vi "Open.vi"(7 "Allow multiple opens?":bool, 8 "error in (no error)":errorcluster, 10 "Channel Names":tag[](array[tag])) -> (0 "error out":errorcluster, 3 "DIO Ref Out":T1)   [LabVIEW 2021, in "DIO.lvlib"]
doc: "Opens a reference to one or more digital I/O channels. You must open a reference before you read or write values."
uses:
  <vilib>/myRIO/Instrument Drivers/Onboard IO/DIO/DIO.lvlib
  <vilib>/myRIO/Instrument Drivers/Onboard IO/DIO/typedefs/DIO Reference.ctl
  <vilib>/myRIO/Common/Instrument Driver Framework/Utilities/typedefs/myRIO Generic Hardware Reference.ctl
  <vilib>/myRIO/Common/Instrument Driver Framework/Utilities/typedefs/Hardware Version Enum.ctl
  <vilib>/myRIO/Common/Instrument Driver Framework/Utilities/typedefs/myRIO v1.0 Reference.ctl
  <vilib>/myRIO/Common/Instrument Driver Framework/Utilities/typedefs/Generic FPGA Reference.ctl
  <vilib>/myRIO/Common/Instrument Driver Framework/myRIO v1.0/DIO/typedefs/DIO Channels List.ctl
  <vilib>/myRIO/Common/Instrument Driver Framework/myRIO v1.0/DIO/typedefs/DIO Channels Enum.ctl
  <vilib>/myRIO/Common/Instrument Driver Framework/Utilities/vis/Validate Channels.vi
  <vilib>/myRIO/Common/Instrument Driver Framework/myRIO v1.0/DIO/vis/myRIO v1.0 Reserve DIO.vi
  <vilib>/myRIO/Common/Instrument Driver Framework/roboRIO v1.0/DIO/vis/roboRIO v1.0 Reserve DIO.vi
  <vilib>/myRIO/Common/Instrument Driver Framework/ELVIS III v1.0/DIO/vis/ELVIS III v1.0 Reserve DIO.vi
  <vilib>/myRIO/Common/Instrument Driver Framework/myRIO v1.0/Resource Manager/vis/myRIO v1.0 Reserve Channel List.vi
  <vilib>/myRIO/Common/Instrument Driver Framework/myRIO v1.0/DIO/vis/myRIO v1.0 Build MUX Configuration DIO.vi
  <vilib>/myRIO/Common/Instrument Driver Framework/roboRIO v1.0/DIO/vis/roboRIO v1.0 Build MUX Configuration DIO.vi
  <vilib>/myRIO/Common/Instrument Driver Framework/roboRIO v1.0/Resource Manager/vis/roboRIO v1.0 Reserve Channel List.vi
  <vilib>/myRIO/Common/Instrument Driver Framework/ELVIS III v1.0/DIO/vis/ELVIS III v1.0 Build MUX Configuration DIO.vi
  <vilib>/myRIO/Common/Instrument Driver Framework/myRIO v1.0/Resource Manager/vis/myRIO v1.0 Reserve Channel.vi
  <vilib>/myRIO/Common/Instrument Driver Framework/myRIO v1.0/Resource Manager/vis/myRIO v1.0 Unreserve Channel.vi
  <vilib>/myRIO/Common/Instrument Driver Framework/myRIO v1.0/Resource Manager/vis/myRIO v1.0 Create Configuration List.vi
  <vilib>/myRIO/Common/Instrument Driver Framework/roboRIO v1.0/Resource Manager/vis/roboRIO v1.0 Create Configuration List.vi
  <vilib>/myRIO/Common/Instrument Driver Framework/roboRIO v1.0/Resource Manager/vis/roboRIO v1.0 Reserve Channel.vi
  <vilib>/myRIO/Common/Instrument Driver Framework/roboRIO v1.0/Resource Manager/vis/roboRIO v1.0 Unreserve Channel.vi
  <vilib>/myRIO/Common/Instrument Driver Framework/ELVIS III v1.0/Resource Manager/vis/ELVIS III v1.0 Create Configuration List.vi
  <vilib>/myRIO/Common/Instrument Driver Framework/myRIO v1.0/Resource Manager/vis/myRIO v1.0 Build Mutex Name.vi
  <vilib>/myRIO/Common/Instrument Driver Framework/roboRIO v1.0/Resource Manager/vis/roboRIO v1.0 Build Mutex Name.vi
  <vilib>/Utility/VariantDataType/GetNumericInfo.vi
  <vilib>/myRIO/Common/Instrument Driver Framework/Utilities/vis/IO Manager.vi
  <vilib>/myRIO/Common/Instrument Driver Framework/Utilities/vis/Configuration Manager.vi
  <vilib>/myRIO/Common/Instrument Driver Framework/myRIO v1.0/Resource Manager/vis/myRIO v1.0 Configure IO.vi
  <vilib>/myRIO/Common/Instrument Driver Framework/myRIO v1.0/myRIO v1.0 Close.vi
  <vilib>/myRIO/Common/Instrument Driver Framework/roboRIO v1.0/Resource Manager/vis/roboRIO v1.0 Configure IO.vi
  <vilib>/myRIO/Common/Instrument Driver Framework/ELVIS III v1.0/Resource Manager/vis/ELVIS III v1.0 Reserve Channel List.vi
  <vilib>/myRIO/Common/Instrument Driver Framework/ELVIS III v1.0/Resource Manager/vis/ELVIS III v1.0 Configure IO.vi
  <vilib>/userdefined/High Color/nirio_resource_hc.ctl
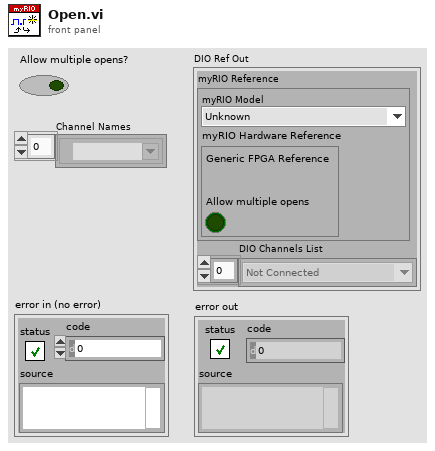
[diagram p1: front panel]
types:
  T1 = typedef "DIO.lvlib/DIO Reference.ctl" = cluster{"myRIO Reference":T2, "DIO Channels List":T6}
  T2 = typedef "myRIO Generic Hardware Reference.ctl" = cluster{"myRIO Model":T3, "myRIO Hardware Reference":T4}
  T3 = typedef "Hardware Version Enum.ctl" = enum16{"Unknown", "myRIO-1900", "myRIO-1950", "roboRIO", "NI ELVIS RIO CM", "ELVIS III"}
  T4 = typedef "myRIO v1.0 Reference.ctl" = cluster{"Generic FPGA Reference":T5, "Allow multiple opens":bool}
  T5 = typedef "Generic FPGA Reference.ctl" = refnum<k20>
  T6 = typedef "DIO Channels List.ctl" = T7[]
  T7 = typedef "DIO Channels Enum.ctl" = enum16{"Not Connected", "C/DIO0", "C/DIO1", "C/DIO2", "C/DIO3", "C/DIO4", "C/DIO5", "C/DIO6", "C/DIO7", "A/DIO0", "A/DIO1", "A/DIO2", "A/DIO3", "A/DIO4", "A/DIO5", "A/DIO6", "A/DIO7", "A/DIO8", "A/DIO9", "A/DIO10", "A/DIO11", "A/DIO12", "A/DIO13", "A/DIO14", "A/DIO15", "A/DIO16", "A/DIO17", "A/DIO18", "A/DIO19", "B/DIO0", "B/DIO1", "B/DIO2", "B/DIO3", "B/DIO4", "B/DIO5", "B/DIO6", "B/DIO7", "B/DIO8", "B/DIO9", "B/DIO10", "B/DIO11", "B/DIO12", "B/DIO13", "B/DIO14", "B/DIO15", "B/DIO16", "B/DIO17", "B/DIO18", "B/DIO19", "LED0", "LED1", "LED2", "LED3", "Button0", "DIO/DIO0", "DIO/DIO1", "DIO/DIO2", "DIO/DIO3", "DIO/DIO4", "DIO/DIO5", "DIO/DIO6", "DIO/DIO7", "DIO/DIO8", "DIO/DIO9", "SPI/CS0", "SPI/CS1", "SPI/CS2", "SPI/CS3", "LED RADIO (Green)", "LED RADIO (Red)", "LED COMM (Green)", "LED COMM (Red)", "LED MODE (Green)", "LED MODE (Red)"}
  T8 = typedef "nirio_resource_hc.ctl" = tag
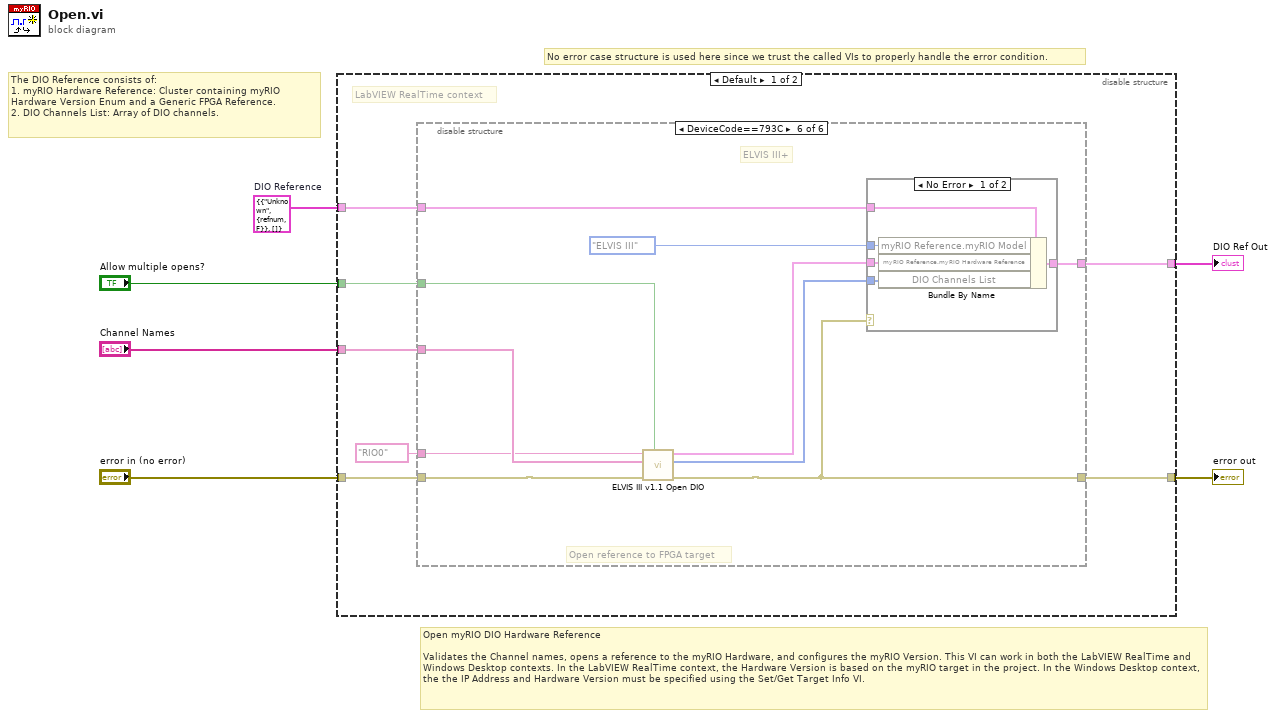
[diagram p0: block diagram]
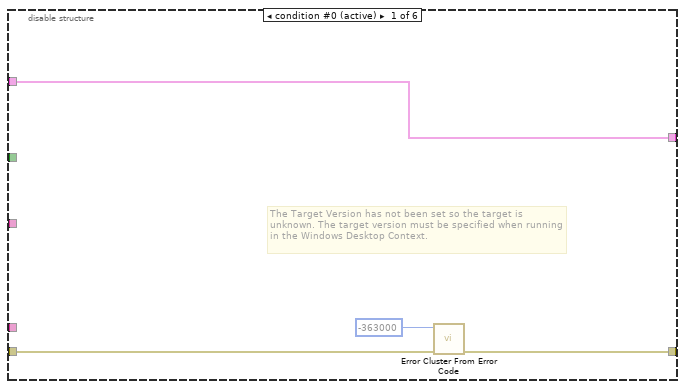
[diagram p2: hidden frame]
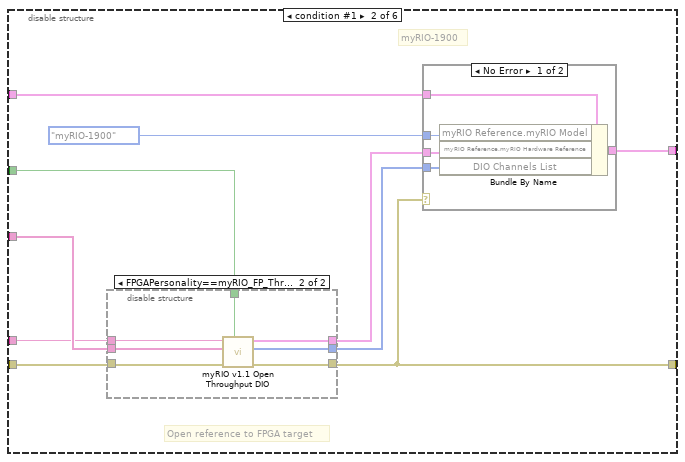
[diagram p3: hidden frame]
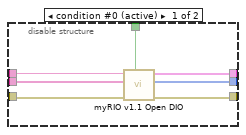
[diagram p4: hidden frame]
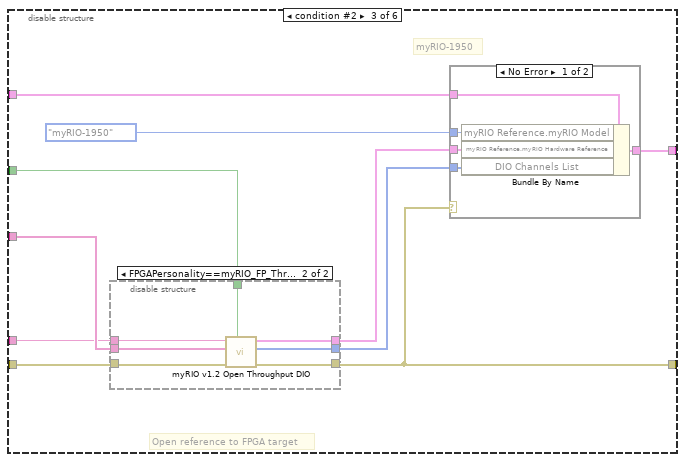
[diagram p6: hidden frame]
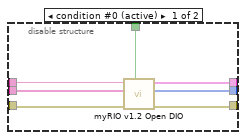
[diagram p7: hidden frame]
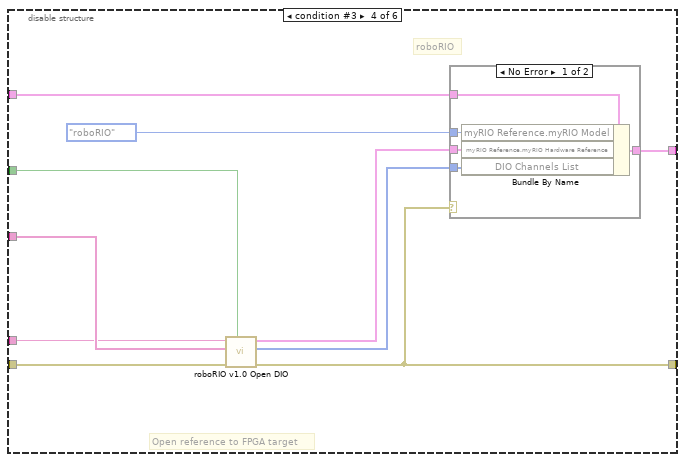
[diagram p9: hidden frame]
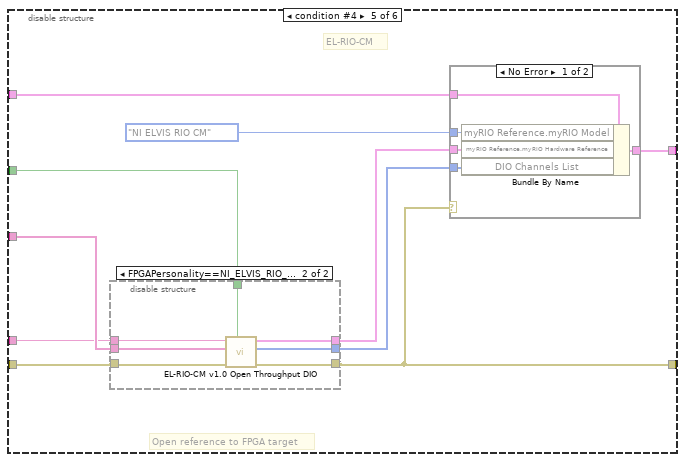
[diagram p11: hidden frame]
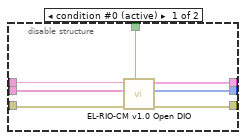
[diagram p12: hidden frame]
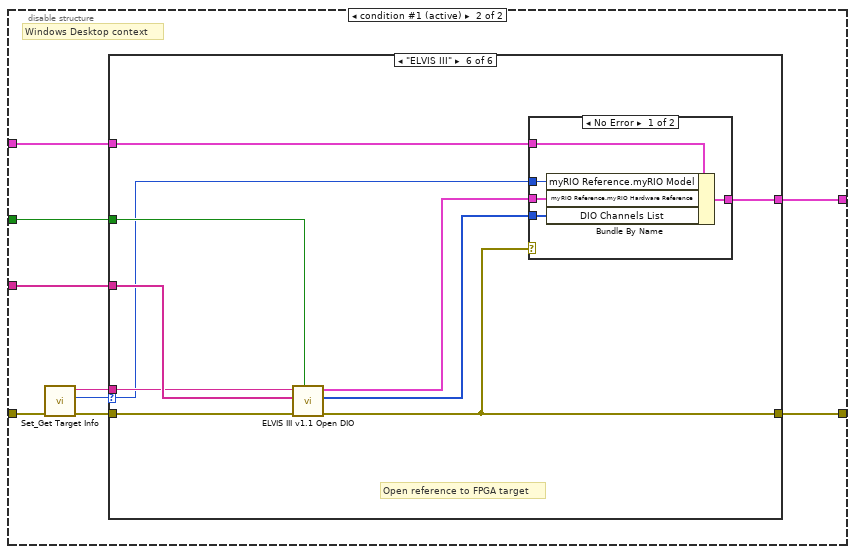
[diagram p15: hidden frame]
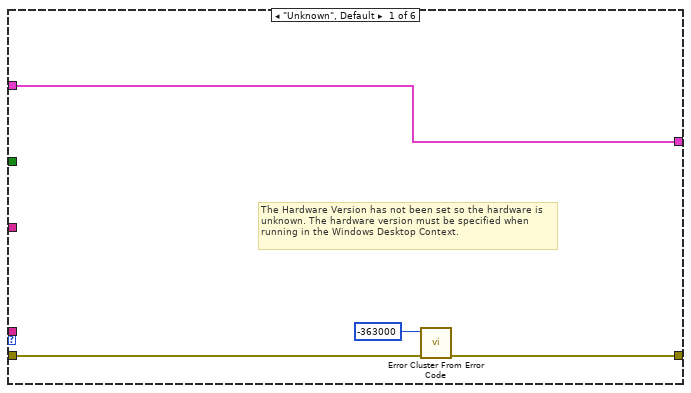
[diagram p16: hidden frame]
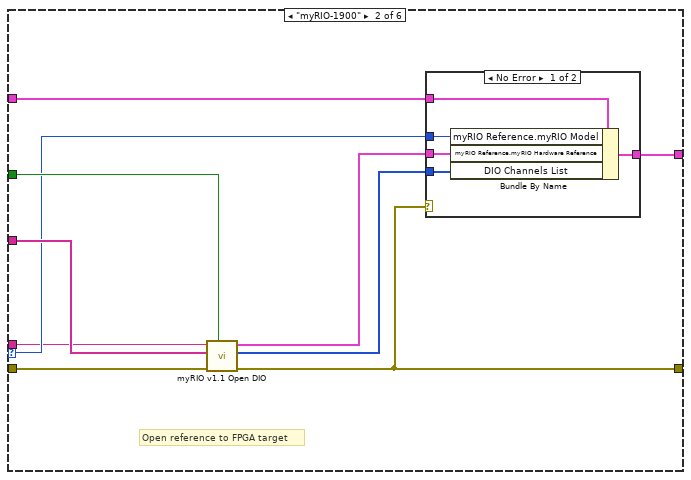
[diagram p17: hidden frame]
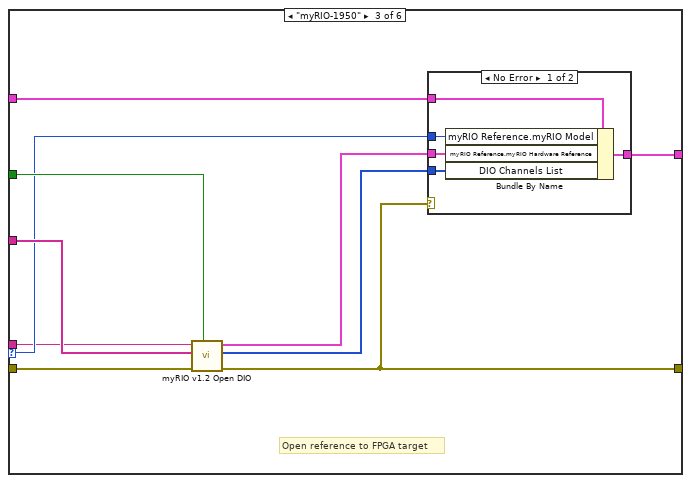
[diagram p19: hidden frame]
diagram:
  w3 = T1 {"myRIO Reference"={"myRIO Model"=enum."Unknown", "myRIO Hardware Reference"={"Generic FPGA Reference"=refnum, "Allow multiple opens"=FALSE}}, "DIO Channels List"=[]}  # DIO Reference
  # "Open myRIO DIO Hardware Reference\n\nValidates the Channel names, opens a reference to the myRIO Hardware, and configures the myRIO Version. This VI can work in both the LabVIEW RealTime and Windows Desktop contexts. In the LabVIEW RealTime context, the Hardware Version is based on the myRIO target in the project. In the Windows Desktop context, the the IP Address and Hardware Version must be specified using the Set/Get Target Info VI."
  # "No error case structure is used here since we trust the called VIs to properly handle the error condition."
  # "The DIO Reference consists of:\n1. myRIO Hardware Reference: Cluster containing myRIO Hardware Version Enum and a Generic FPGA Reference.\n2. DIO Channels List: Array of DIO channels."
  n1 = disable-structure shown="Default" {
    disable-tunnel: [w13 w147] -> w6
    disable-tunnel: "Channel Names" -> [w12 w144]
    disable-tunnel: "Allow multiple opens?" -> [w11 w146]
    disable-tunnel: [w10 w145] -> w2
    disable-tunnel: "error in (no error)" -> [w9 w143]
    disable-tunnel: w3 -> [w8 w142]
    frame condition #0 {
      # "LabVIEW RealTime context"
      n2 = disable-structure shown="DeviceCode==793C" {
        disable-tunnel: [w17 w18 w48 w78 w100 w125] -> w13
        disable-tunnel: w12 -> [_ w27 w57 w87 w96 w128]
        disable-tunnel: w11 -> [_ w22 w56 w86 w94 w129]
        disable-tunnel: [w14 w26 w55 w85 w103 w124] -> w10
        disable-tunnel: w9 -> [w16 w24 w53 w83 w97 w126]
        disable-tunnel: w8 -> [w14 w21 w51 w81 w101 w130]
        disable-tunnel: T8 "RIO0" ("Resource name") -> [_ w19 w49 w79 w95 w127]
        frame condition #0 (active) {
          # "The Target Version has not been set so the target is unknown. The target version must be specified when running in the Windows Desktop Context."
          n3 = call <vilib>:"Error Cluster From Error Code.vi"("error in (no error)"=w16, "error code (0)"=-363000) -> ("error out"=w17:errorcluster)  [unwired: 7 in]
        }
        frame condition #1 {
          # "myRIO-1900"
          # "Open reference to FPGA target"
          n4 = disable-structure shown="FPGAPersonality==myRIO_FP_Throughput" {
            disable-tunnel: w27 -> [w34 w41]
            disable-tunnel: w24 -> [w33 w40]
            disable-tunnel: [w32 w39] -> w23
            disable-tunnel: w22 -> [w31 w38]
            disable-tunnel: [w30 w37] -> w20
            disable-tunnel: w19 -> [w29 w36]
            disable-tunnel: [w28 w35] -> w18
            frame condition #0 (active) {
              n5 = call <vilib>:"myRIO v1.1 Open DIO.vi"("Allow multiple opens?"=w31, "error in (no error)"=w33, "Channel Names"=w34, "Resource name"=w29) -> ("error out"=w28:errorcluster, "DIO Channel List"=w30:T6, "myRIO Ref Out"=w32:T4)  [unwired: 5 in]
            }
            frame condition #1 {
              n6 = call <vilib>:"myRIO v1.1 Open Throughput DIO.vi"("Allow multiple opens?"=w38, "error in (no error)"=w40, "Channel Names"=w41, "Resource name"=w36) -> ("error out"=w35:errorcluster, "DIO Channel List"=w37:T6, "myRIO Ref Out"=w39:T4)  [unwired: 5 in]
            }
          }
          n7 = case shown="No Error" w18 {
            tunnel: [w46 w47] -> w26
            tunnel: Hardware_Version_Enum."myRIO-1900" ("Hardware Version Enum") -> [w45 _]
            tunnel: w23 -> [w42 _]
            tunnel: w21 -> [w44 w47]
            tunnel: w20 -> [w43 _]
            frame No Error {
              n8 = Bundle By Name(cluster=w44, "myRIO Reference.myRIO Model"=w45, "myRIO Reference.myRIO Hardware Reference"=w42, "DIO Channels List"=w43) -> (w46:T1)
            }
            frame Error {
            }
          }
        }
        frame condition #2 {
          # "myRIO-1950"
          # "Open reference to FPGA target"
          n9 = disable-structure shown="FPGAPersonality==myRIO_FP_Throughput" {
            disable-tunnel: w57 -> [w64 w71]
            disable-tunnel: w56 -> [w63 w70]
            disable-tunnel: w53 -> [w62 w69]
            disable-tunnel: [w61 w68] -> w52
            disable-tunnel: [w60 w67] -> w50
            disable-tunnel: w49 -> [w59 w66]
            disable-tunnel: [w58 w65] -> w48
            frame condition #0 (active) {
              n10 = call <vilib>:"myRIO v1.2 Open DIO.vi"("Allow multiple opens?"=w63, "error in (no error)"=w62, "Channel Names"=w64, "Resource name"=w59) -> ("error out"=w58:errorcluster, "DIO Channel List"=w60:T6, "myRIO Ref Out"=w61:T4)  [unwired: 5 in]
            }
            frame condition #1 {
              n11 = call <vilib>:"myRIO v1.2 Open Throughput DIO.vi"("Allow multiple opens?"=w70, "error in (no error)"=w69, "Channel Names"=w71, "Resource name"=w66) -> ("error out"=w65:errorcluster, "DIO Channel List"=w67:T6, "myRIO Ref Out"=w68:T4)  [unwired: 5 in]
            }
          }
          n12 = case shown="No Error" w48 {
            tunnel: [w76 w77] -> w55
            tunnel: Hardware_Version_Enum."myRIO-1950" ("Hardware Version Enum") -> [w75 _]
            tunnel: w52 -> [w74 _]
            tunnel: w51 -> [w73 w77]
            tunnel: w50 -> [w72 _]
            frame No Error {
              n13 = Bundle By Name(cluster=w73, "myRIO Reference.myRIO Model"=w75, "myRIO Reference.myRIO Hardware Reference"=w74, "DIO Channels List"=w72) -> (w76:T1)
            }
            frame Error {
            }
          }
        }
        frame condition #3 {
          # "roboRIO"
          # "Open reference to FPGA target"
          n14 = call <vilib>:"roboRIO v1.0 Open DIO.vi"("Allow multiple opens?"=w86, "error in (no error)"=w83, "Channel Names"=w87, "Resource name"=w79) -> ("error out"=w78:errorcluster, "DIO Channel List"=w80:T6, "myRIO Ref Out"=w82:T4)  [unwired: 5 in]
          n15 = case shown="No Error" w78 {
            tunnel: [w92 w93] -> w85
            tunnel: Hardware_Version_Enum."roboRIO" ("Hardware Version Enum") -> [w91 _]
            tunnel: w82 -> [w90 _]
            tunnel: w81 -> [w89 w93]
            tunnel: w80 -> [w88 _]
            frame No Error {
              n16 = Bundle By Name(cluster=w89, "myRIO Reference.myRIO Model"=w91, "myRIO Reference.myRIO Hardware Reference"=w90, "DIO Channels List"=w88) -> (w92:T1)
            }
            frame Error {
            }
          }
        }
        frame condition #4 {
          # "EL-RIO-CM"
          # "Open reference to FPGA target"
          n17 = disable-structure shown="FPGAPersonality==NI_ELVIS_RIO_CM_FP_Throughput" {
            disable-tunnel: w96 -> [w110 w112]
            disable-tunnel: w94 -> [w109 w117]
            disable-tunnel: w97 -> [w108 w113]
            disable-tunnel: [w107 w116] -> w98
            disable-tunnel: [w106 w115] -> w99
            disable-tunnel: w95 -> [w105 w111]
            disable-tunnel: [w104 w114] -> w100
            frame condition #0 (active) {
              n18 = call <vilib>:"EL-RIO-CM v1.0 Open DIO.vi"("Allow multiple opens?"=w109, "error in (no error)"=w108, "Channel Names"=w110, "Resource name"=w105) -> ("error out"=w104:errorcluster, "DIO Channel List"=w106:T6, "myRIO Ref Out"=w107:T4)  [unwired: 5 in]
            }
            frame condition #1 {
              n19 = call <vilib>:"EL-RIO-CM v1.0 Open Throughput DIO.vi"("Allow multiple opens?"=w117, "error in (no error)"=w113, "Channel Names"=w112, "Resource name"=w111) -> ("error out"=w114:errorcluster, "DIO Channel List"=w115:T6, "myRIO Ref Out"=w116:T4)  [unwired: 5 in]
            }
          }
          n20 = case shown="No Error" w100 {
            tunnel: [w122 w123] -> w103
            tunnel: Hardware_Version_Enum."NI ELVIS RIO CM" ("Hardware Version Enum") -> [w121 _]
            tunnel: w98 -> [w120 _]
            tunnel: w101 -> [w119 w123]
            tunnel: w99 -> [w118 _]
            frame No Error {
              n21 = Bundle By Name(cluster=w119, "myRIO Reference.myRIO Model"=w121, "myRIO Reference.myRIO Hardware Reference"=w120, "DIO Channels List"=w118) -> (w122:T1)
            }
            frame Error {
            }
          }
        }
        frame condition #5 {
          # "ELVIS III+"
          # "Open reference to FPGA target"
          n22 = call <vilib>:"ELVIS III v1.1 Open DIO.vi"("Allow multiple opens?"=w129, "error in (no error)"=w126, "Channel Names"=w128, "Resource name"=w127) -> ("error out"=w125:errorcluster, "DIO Channel List"=w132:T6, "myRIO Ref Out"=w131:T4)  [unwired: 5 in]
          n23 = case shown="No Error" w125 {
            tunnel: [w138 w139] -> w124
            tunnel: Hardware_Version_Enum."ELVIS III" ("Hardware Version Enum") -> [w137 _]
            tunnel: w131 -> [w136 _]
            tunnel: w130 -> [w135 w139]
            tunnel: w132 -> [w134 _]
            frame No Error {
              n24 = Bundle By Name(cluster=w135, "myRIO Reference.myRIO Model"=w137, "myRIO Reference.myRIO Hardware Reference"=w136, "DIO Channels List"=w134) -> (w138:T1)
            }
            frame Error {
            }
          }
        }
      }
    }
    frame condition #1 (active) {
      # "Windows Desktop context"
      n25 = call <vilib>:"Set_Get Target Info.vi"() -> ("Hardware Version"=w140:T3, "IP Address"=w141:string)  [unwired: 9 in, 1 out]
      n26 = case shown="\"ELVIS III\"" w140 {
        selector: w140 -> [_ w157 w174 w190 w206 w219]
        tunnel: [w151 w152 w168 w184 w200 w217] -> w147
        tunnel: w144 -> [_ w161 w177 w193 w209 w221]
        tunnel: w146 -> [_ w160 w176 w192 w208 w222]
        tunnel: [w148 w159 w169 w185 w201 w216] -> w145
        tunnel: w143 -> [w149 w153 w173 w189 w205 w218]
        tunnel: w141 -> [_ w156 w172 w188 w204 w220]
        tunnel: w142 -> [w148 w155 w171 w187 w203 w223]
        frame "Unknown", Default {
          # "The Hardware Version has not been set so the hardware is unknown. The hardware version must be specified when running in the Windows Desktop Context."
          n27 = call <vilib>:"Error Cluster From Error Code.vi"("error in (no error)"=w149, "error code (0)"=-363000) -> ("error out"=w151:errorcluster)  [unwired: 7 in]
        }
        frame "myRIO-1900" {
          # "Open reference to FPGA target"
          n28 = call <vilib>:"myRIO v1.1 Open DIO.vi"("Allow multiple opens?"=w160, "error in (no error)"=w153, "Channel Names"=w161, "Resource name"=w156) -> ("error out"=w152:errorcluster, "DIO Channel List"=w154:T6, "myRIO Ref Out"=w158:T4)  [unwired: 5 in]
          n29 = case shown="No Error" w152 {
            tunnel: [w166 w167] -> w159
            tunnel: w158 -> [w165 _]
            tunnel: w157 -> [w164 _]
            tunnel: w155 -> [w163 w167]
            tunnel: w154 -> [w162 _]
            frame No Error {
              n30 = Bundle By Name(cluster=w163, "myRIO Reference.myRIO Model"=w164, "myRIO Reference.myRIO Hardware Reference"=w165, "DIO Channels List"=w162) -> (w166:T1)
            }
            frame Error {
            }
          }
        }
        frame "myRIO-1950" {
          # "Open reference to FPGA target"
          n31 = call <vilib>:"myRIO v1.2 Open DIO.vi"("Allow multiple opens?"=w176, "error in (no error)"=w173, "Channel Names"=w177, "Resource name"=w172) -> ("error out"=w168:errorcluster, "DIO Channel List"=w170:T6, "myRIO Ref Out"=w175:T4)  [unwired: 5 in]
          n32 = case shown="No Error" w168 {
            tunnel: w175 -> [w182 _]
            tunnel: w174 -> [w181 _]
            tunnel: w171 -> [w180 w183]
            tunnel: w170 -> [w179 _]
            tunnel: [w178 w183] -> w169
            frame No Error {
              n33 = Bundle By Name(cluster=w180, "myRIO Reference.myRIO Model"=w181, "myRIO Reference.myRIO Hardware Reference"=w182, "DIO Channels List"=w179) -> (w178:T1)
            }
            frame Error {
            }
          }
        }
        frame "roboRIO" {
          # "Open reference to FPGA target"
          n34 = call <vilib>:"roboRIO v1.0 Open DIO.vi"("Allow multiple opens?"=w192, "error in (no error)"=w189, "Channel Names"=w193, "Resource name"=w188) -> ("error out"=w184:errorcluster, "DIO Channel List"=w186:T6, "myRIO Ref Out"=w191:T4)  [unwired: 5 in]
          n35 = case shown="No Error" w184 {
            tunnel: w191 -> [w198 _]
            tunnel: w190 -> [w197 _]
            tunnel: w187 -> [w196 w199]
            tunnel: w186 -> [w195 _]
            tunnel: [w194 w199] -> w185
            frame No Error {
              n36 = Bundle By Name(cluster=w196, "myRIO Reference.myRIO Model"=w197, "myRIO Reference.myRIO Hardware Reference"=w198, "DIO Channels List"=w195) -> (w194:T1)
            }
            frame Error {
            }
          }
        }
        frame "NI ELVIS RIO CM" {
          # "Open reference to FPGA target"
          n37 = call <vilib>:"EL-RIO-CM v1.0 Open DIO.vi"("Allow multiple opens?"=w208, "error in (no error)"=w205, "Channel Names"=w209, "Resource name"=w204) -> ("error out"=w200:errorcluster, "DIO Channel List"=w202:T6, "myRIO Ref Out"=w207:T4)  [unwired: 5 in]
          n38 = case shown="No Error" w200 {
            tunnel: w207 -> [w214 _]
            tunnel: w206 -> [w213 _]
            tunnel: w203 -> [w212 w215]
            tunnel: w202 -> [w211 _]
            tunnel: [w210 w215] -> w201
            frame No Error {
              n39 = Bundle By Name(cluster=w212, "myRIO Reference.myRIO Model"=w213, "myRIO Reference.myRIO Hardware Reference"=w214, "DIO Channels List"=w211) -> (w210:T1)
            }
            frame Error {
            }
          }
        }
        frame "ELVIS III" {
          # "Open reference to FPGA target"
          n40 = call <vilib>:"ELVIS III v1.1 Open DIO.vi"("Allow multiple opens?"=w222, "error in (no error)"=w218, "Channel Names"=w221, "Resource name"=w220) -> ("error out"=w217:errorcluster, "DIO Channel List"=w224:T6, "myRIO Ref Out"=w225:T4)  [unwired: 5 in]
          n41 = case shown="No Error" w217 {
            tunnel: w225 -> [w230 _]
            tunnel: w219 -> [w229 _]
            tunnel: w223 -> [w228 w231]
            tunnel: w224 -> [w227 _]
            tunnel: [w226 w231] -> w216
            frame No Error {
              n42 = Bundle By Name(cluster=w228, "myRIO Reference.myRIO Model"=w229, "myRIO Reference.myRIO Hardware Reference"=w230, "DIO Channels List"=w227) -> (w226:T1)
            }
            frame Error {
            }
          }
        }
      }
    }
  }
  "DIO Ref Out" <- w2
  "error out" <- w6
